vi "Get Pump Power.vi"(8 "error in (no error)":errorcluster, 11 "VISA session":refnum<visa-resource-name>) -> (0 "error out":errorcluster, 1 "Pump Speed":i32, 2 "Returned String":string, 3 "dup VISA session":refnum<visa-resource-name>)   [LabVIEW 2018, in "Lauda TCU.lvlib"]
uses:
  Lauda TCU.lvlib
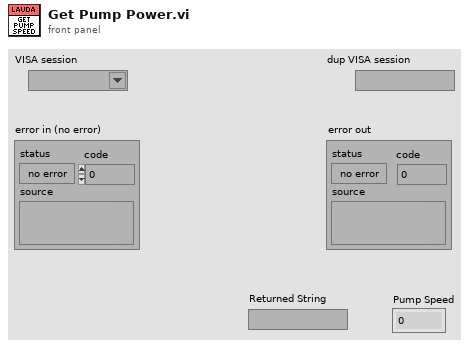
[diagram p1: front panel]
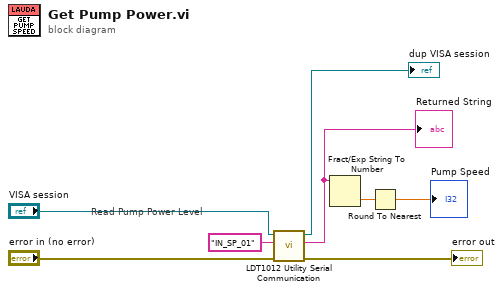
[diagram p0: block diagram]
diagram:
  # "Read Pump Power Level"
  n1 = call "LDT1012 Utility Serial Communication.vi"("error in (no error)"="error in (no error)", "Command String"="IN_SP_01", "VISA session"="VISA session") -> ("error out"=→"error out":errorcluster, "Returned String"=w3:string, "dup VISA session"=→"dup VISA session":refnum<visa-resource-name>)  [unwired: 5 in, 1 out]
  "Returned String" <- w3
  n2 = Fract/Exp String To Number(string=w3) -> (number=w2:dbl)  [unwired: 3 in, 1 out]
  n3 = Round To Nearest(number=w2) -> (nearest integer value=→"Pump Speed":dbl)
